vi "Lecture Param Sys.vi"(8 "errin":errorcluster) -> (0 "error out":errorcluster caption="errout")   [LabVIEW 2020]
uses:
  <vilib>/Utility/config.llb/Read Key (Double).vi
  <vilib>/Utility/config.llb/Read Key (String).vi
  Param_Sys.vi
  <vilib>/Utility/config.llb/NI_LVConfig.lvlib
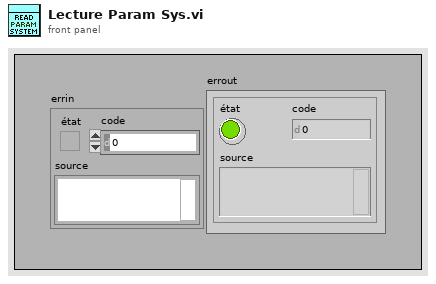
[diagram p1: front panel]
types:
  T1 = typedef "NI_LVConfig.lvlib/Config Data RefNum.ctl" = refnum<k1>
  T2 = cluster{"[0]":string, "[1]":string, "[2]":string, "[3]":string, "[4]":string}
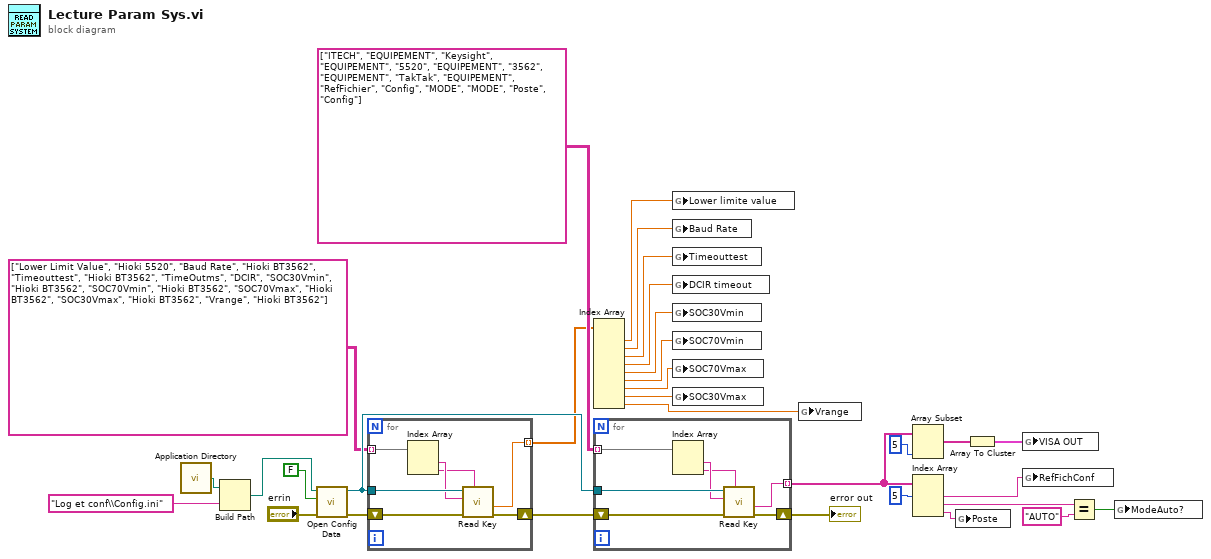
[diagram p0: block diagram]
diagram:
  n1 = call <vilib>:"Application Directory.vi"() -> ("Application Directory"=w26:path)
  n2 = Build Path(base path=w26, name or relative path="Log et conf\\Config.ini") -> (appended path=w30:path)
  n3 = call <vilib>:"Open Config Data.vi"("error in (no error)"="errin", "create file if necessary (T)"=FALSE, "configuration file path"=w30) -> ("error out"=w28:errorcluster, "refnum"=w23:T1)  [unwired: 6 in, 1 out]
  n4 = for {
    tunnel: w23 -> [w37]
    tunnel: string[][] [["Lower Limit Value", "Hioki 5520"], ["Baud Rate", "Hioki BT3562"], ["Timeouttest", "Hioki BT3562"], ["TimeOutms", "DCIR"], ["SOC30Vmin", "Hioki BT3562"], ["SOC70Vmin", "Hioki BT3562"], ["SOC70Vmax", "Hioki BT3562"], ["SOC30Vmax", "Hioki BT3562"], ["Vrange", "Hioki BT3562"]] -> [w36] mode=indexing
    shift-right: [w33] -> w25
    shift-left: w28 -> [w38]
    tunnel: [w32] -> w14 mode=indexing
    n5 = Index Array(array=w36) -> (element #1=w35:string, element #2=w34:string)  [unwired: 2 in]
    n6 = call-poly <vilib>:"Read Key.vi"("section"=w34, "error in (no error)"=w38, "key"=w35, "refnum"=w37) -> ("error out"=w33:errorcluster, "value"=w32:dbl)  [unwired: 4 in, 2 out]
  }
  n7 = Index Array(array=w14) -> (element #1=w13:dbl, element #2=w12:dbl, element #3=w11:dbl, element #4=w10:dbl, element #5=w9:dbl, element #6=w8:dbl, element #7=w7:dbl, element #8=w6:dbl, element #9=w1:dbl)  [unwired: 9 in]
  n8 = for {
    tunnel: w23 -> [w44]
    tunnel: string[][] [["ITECH", "EQUIPEMENT"], ["Keysight", "EQUIPEMENT"], ["5520", "EQUIPEMENT"], ["3562", "EQUIPEMENT"], ["TakTak", "EQUIPEMENT"], ["RefFichier", "Config"], ["MODE", "MODE"], ["Poste", "Config"]] -> [w43] mode=indexing
    shift-right: [w40] -> w24
    shift-left: w25 -> [w45]
    tunnel: [w39] -> w19 mode=indexing
    n9 = Index Array(array=w43) -> (element #1=w42:string, element #2=w41:string)  [unwired: 2 in]
    n10 = call-poly <vilib>:"Read Key.vi"("section"=w41, "error in (no error)"=w45, "key"=w42, "refnum"=w44) -> ("error out"=w40:errorcluster, "value"=w39:string)  [unwired: 4 in, 2 out]
  }
  "error out" <- w24
  n11 = global write "Param_Sys.vi" "Lower limite value"(w13) -> ()
  n12 = global write "Param_Sys.vi" "Baud Rate"(w12) -> ()
  n13 = global write "Param_Sys.vi" "Timeouttest"(w11) -> ()
  n14 = global write "Param_Sys.vi" "DCIR timeout"(w10) -> ()
  n15 = global write "Param_Sys.vi" "SOC30Vmin"(w9) -> ()
  n16 = global write "Param_Sys.vi" "SOC70Vmin"(w8) -> ()
  n17 = global write "Param_Sys.vi" "SOC70Vmax"(w7) -> ()
  n18 = global write "Param_Sys.vi" "SOC30Vmax"(w6) -> ()
  n19 = global write "Param_Sys.vi" "Vrange"(w1) -> ()
  n20 = Array Subset(array=w19, length=5 ("longueur")) -> (w22:string[])  [unwired: 1 in]
  n21 = Index Array(array=w19, index #1=5 ("indice")) -> (element #1=w4:string, element #2=w18:string, element #3=w2:string)  [unwired: 2 in]
  n22 = global write "Param_Sys.vi" "Poste"(w2) -> ()
  n23 = Array To Cluster(array=w22) -> (cluster=w5:T2)
  n24 = global write "Param_Sys.vi" "VISA OUT"(w5) -> ()
  n25 = global write "Param_Sys.vi" "RefFichConf"(w4) -> ()
  n26 = Equal? ("Égaux ?")(x=w18, y="AUTO") -> (x = y?=w3:bool)
  n27 = global write "Param_Sys.vi" "ModeAuto?"(w3) -> ()
